vi "Test Process within App Log Error Message When Setting Handler After Process.vi"(8 "error in (no error)":errorcluster, 11 "Test Case In":refnum<class "Logger Test.lvclass">) -> (0 "error out":errorcluster, 3 "Test Case Out":refnum<class "Logger Test.lvclass">)   [LabVIEW 2020, in "Logger Test.lvclass"]
uses:
  Logger Test.lvclass
  Logger Test.lvclass/Logger Test.ctl
  source/Framework Test Suite/Mock Log Handler/Mock Log Handler.lvclass
  source/Framework/Process/Process.lvclass
  source/Framework/Logging/Logging.lvclass
  source/Framework/Application/Application.lvclass
  source/Framework Test Suite/Mock Process/Mock Process.lvclass
  source/Framework Test Suite/Support/Test Support.lvlib
  C:/Git/astemes-triarc-framework/source/Framework/Process/Process.lvclass
  C:/Git/astemes-triarc-framework/source/Framework/Base/Base.lvclass
  C:/Git/astemes-triarc-framework/source/Framework/Error Handler Interface/Error Handler Interface.lvclass
  C:/Git/astemes-triarc-framework/source/Framework/Logging/Logging.lvclass
  C:/Git/astemes-triarc-framework/source/Framework/Application/Application.lvclass
  C:/Git/astemes-triarc-framework/source/Framework/Async Handler/Async Handler.lvclass
  07009c05-29cc-44a3-a854-ccf813a5e6df.vi
  C:/Git/astemes-triarc-framework/source/Framework/Configuration File/Configuration File.lvclass
  C:/Git/astemes-triarc-framework/source/Framework/Configuration/Configuration.lvclass
  C:/Git/astemes-triarc-framework/source/Framework Test Suite/Mock Process/Mock Process.lvclass
  C:/Git/astemes-triarc-framework/source/Framework/Helper Loop/Helper Loop.lvclass
  C:/Git/astemes-triarc-framework/source/Framework Test Suite/Mock Log Handler/Mock Log Handler.lvclass
  6e911bec-e8a5-4451-b4a0-22b7fdbbda38.vi
  34049daa-a343-404c-9e84-4ab9e23fdc36.vi
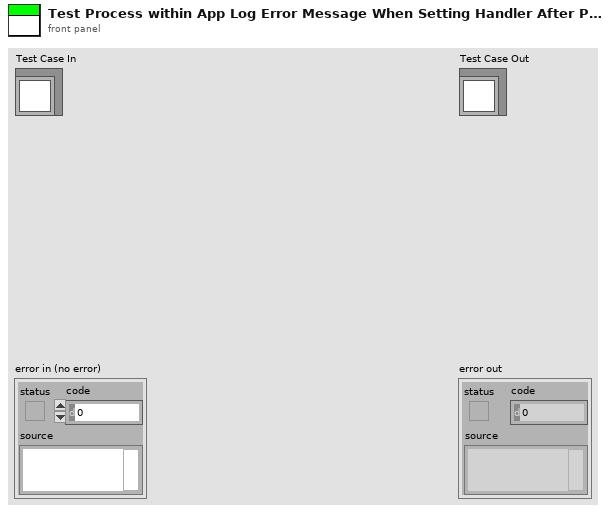
[diagram p1: front panel]
types:
  T1 = typedef "Mock Log Handler.lvclass/Log Entry.ctl" = cluster{"Level":string, "Source":string, "Message":string}
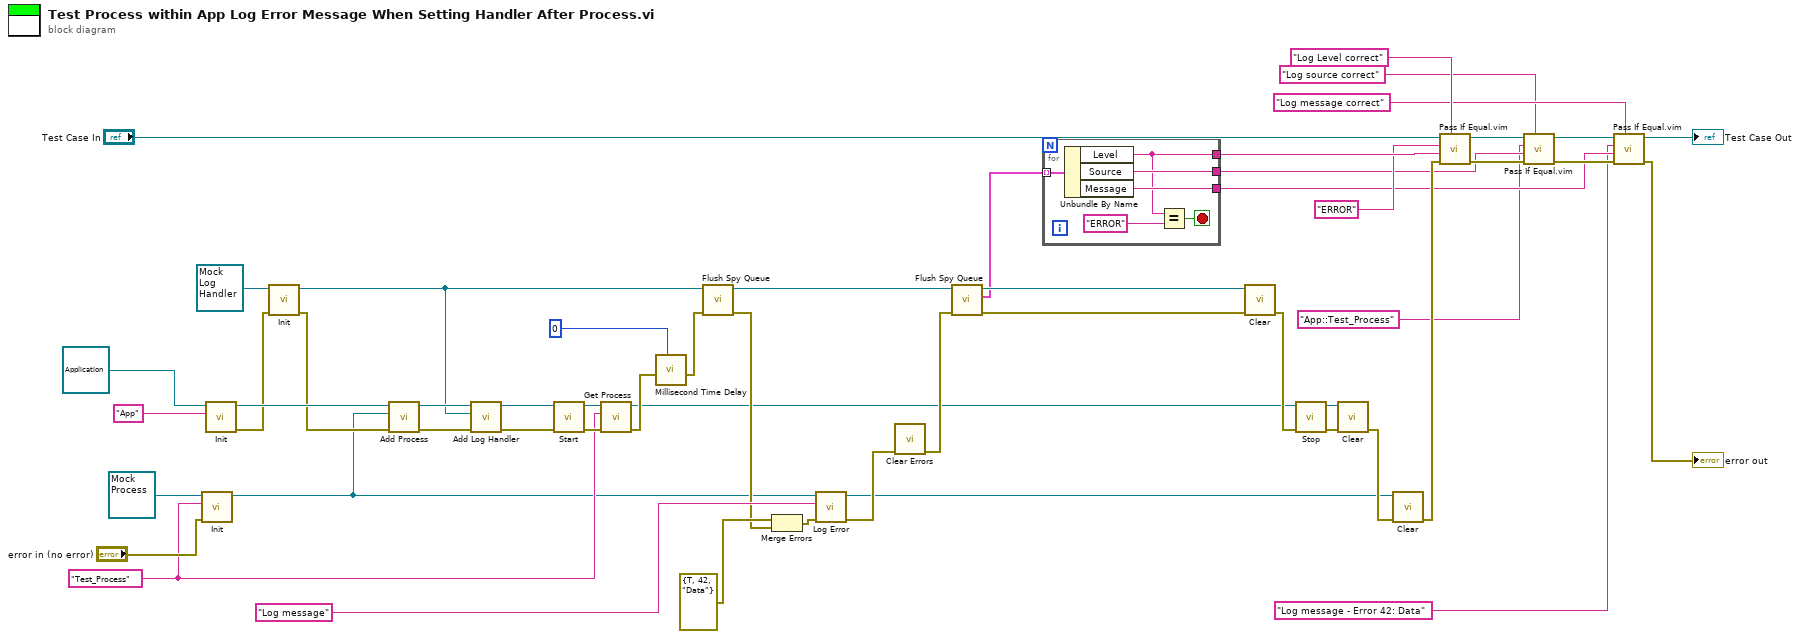
[diagram p0: block diagram]
diagram:
  w3 = "Test_Process" ("Name")
  n1 = call-dynamic "Init.vi"("error in (no error)"="error in (no error)", "Name"=w3, "Mock Process In"=refnum<class "Mock Process.lvclass"> refnum) -> ("Mock Process Out"=w2:refnum<class "Mock Process.lvclass">)  [unwired: 7 in, 1 out]
  n2 = call-dynamic "Init.vi"("Name"="App", "Process In"=refnum<class "Application.lvclass"> refnum ("Application.lvclass")) -> ("error out"=w47:errorcluster, "Process Out"=w50:refnum<class "Application.lvclass">)  [unwired: 8 in]
  n3 = call-dynamic "Init.vi"("error in (no error)"=w47, "Mock Log Handler In"=refnum<class "Mock Log Handler.lvclass"> refnum ("Mock Log Handler.lvclass")) -> ("error out"=w46:errorcluster, "Mock Log Handler Out"=w7:refnum<class "Mock Log Handler.lvclass">)  [unwired: 8 in]
  n4 = call "Add Process.vi"("error in (no error)"=w46, "Process"=w2, "Application In"=w50) -> ("error out"=w20:errorcluster, "Application Out"=w9:refnum<class "Application.lvclass">)  [unwired: 7 in]
  n5 = call "Add Log Handler.vi"("error in (no error)"=w20, "Log Handler"=w7, "Process In"=w9) -> ("error out"=w10:errorcluster, "Process Out"=w8:refnum<class "Application.lvclass">)  [unwired: 7 in]
  n6 = call "Start.vi"("error in (no error)"=w10, "Process In"=w8) -> ("error out"=w14:errorcluster, "Process Out"=w5:refnum<class "Application.lvclass">)  [unwired: 7 in, 1 out]
  n7 = call "Get Process.vi"("error in (no error)"=w14, "Process Name"=w3, "Application In"=w5) -> ("error out"=w6:errorcluster, "Application Out"=w4:refnum<class "Application.lvclass">)  [unwired: 6 in, 1 out]
  n8 = call "Millisecond Time Delay.vi"("milliseconds to wait"=u32 0, "error in (no error)"=w6) -> ("error out"=w12:errorcluster)  [unwired: 7 in]
  n9 = call "Flush Spy Queue.vi"("error in (no error)"=w12, "Mock Log Handler in"=w7) -> ("error out"=w13:errorcluster, "Mock Log Handler out"=w15:refnum<class "Mock Log Handler.lvclass">)  [unwired: 7 in, 1 out]
  n10 = Merge Errors(errorcluster {"status"=TRUE, "code"=42, "source"="Data"} ("error in (no error)"), w13) -> (w17:errorcluster)
  n11 = call "Log Error.vi"("error in (no error)"=w17, "Message"="Log message", "Logging In"=w2) -> ("error out"=w27:errorcluster, "Logging Out"=w1:refnum<class "Mock Process.lvclass">)  [unwired: 7 in]
  n12 = call <vilib>:"Clear Errors.vi"("error in (no error)"=w27) -> ("error out"=w26:errorcluster)  [unwired: 5 in, 1 out]
  n13 = call "Flush Spy Queue.vi"("error in (no error)"=w26, "Mock Log Handler in"=w15) -> ("error out"=w44:errorcluster, "remaining elements"=w42:T1[], "Mock Log Handler out"=w45:refnum<class "Mock Log Handler.lvclass">)  [unwired: 7 in]
  n14 = for {
    tunnel: w42 -> [w59] mode=indexing
    tunnel: [w55] -> w41
    tunnel: [w58] -> w31
    tunnel: [w57] -> w30
    stop <- w54 stop-if-true
    n15 = Unbundle By Name(w59) -> ("Level"=w55:string, "Source"=w58:string, "Message"=w57:string)
    n16 = Equal?(x=w55, y="ERROR") -> (x = y?=w54:bool)
  }
  n17 = call-dynamic "Clear.vi"("error in (no error)"=w44, "Mock Log Handler In"=w45) -> ("error out"=w43:errorcluster)  [unwired: 9 in]
  n18 = call "Stop.vi"("error in (no error)"=w43, "Process In"=w4) -> ("error out"=w19:errorcluster, "Process Out"=w18:refnum<class "Application.lvclass">)  [unwired: 7 in, 1 out]
  n19 = call-dynamic "Clear.vi"("error in (no error)"=w19, "Application In"=w18) -> ("error out"=w49:errorcluster)  [unwired: 9 in]
  n20 = call-dynamic "Clear.vi"("error in (no error)"=w49, "Mock Process In"=w1) -> ("error out"=w35:errorcluster)  [unwired: 9 in]
  n21 = call "Pass If Equal.vim"("Description"="Log Level correct", "error in (no error)"=w35, "Actual"=w41, "Expected"="ERROR", "LUnit Test Case In"="Test Case In") -> ("error out"=w37:errorcluster, "LUnit Test Case Out"=w52:refnum<class "Logger Test.lvclass">)  [unwired: 5 in]
  n22 = call "Pass If Equal.vim"("Description"="Log source correct", "error in (no error)"=w37, "Actual"=w31, "Expected"="App::Test_Process" ("Name"), "LUnit Test Case In"=w52) -> ("error out"=w36:errorcluster, "LUnit Test Case Out"=w39:refnum<class "Logger Test.lvclass">)  [unwired: 5 in]
  n23 = call "Pass If Equal.vim"("Description"="Log message correct", "error in (no error)"=w36, "Actual"=w30, "Expected"="Log message - Error 42: Data" ("Message"), "LUnit Test Case In"=w39) -> ("error out"=→"error out":errorcluster, "LUnit Test Case Out"=→"Test Case Out":refnum<class "Logger Test.lvclass">)  [unwired: 5 in]
